vi "GetType.vi"(8 "error in (no error)":errorcluster, 11 "Set Output Value Msg":refnum<class "Set Output Value Msg.lvclass">) -> (0 "error out":errorcluster, 2 "Data Sample":variant, 3 "Set Output Value Msg":refnum<class "Set Output Value Msg.lvclass">)   [LabVIEW 2021, in "BNT_ULx.lvlib" / "Set Output Value Msg.lvclass"]
uses:
  Set Output Value Msg.lvclass
  Set Output Value Msg.lvclass/Set Output Value Msg.ctl
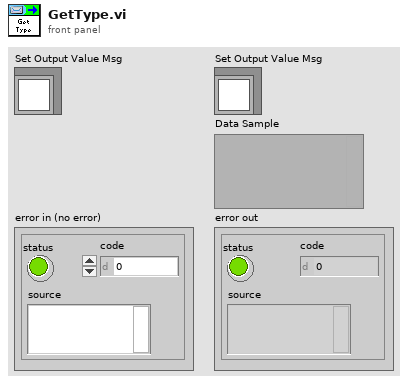
[diagram p1: front panel]
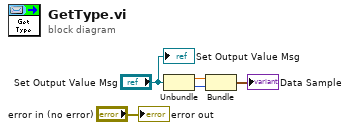
[diagram p0: block diagram]
diagram:
  n1 = Unbundle("Set Output Value Msg") -> (w2:dbl, w1:i32)
  n2 = Bundle("Value"=w2, "Channel"=w1) -> (→"Data Sample":cluster{"Value":dbl, "Channel":i32})  [unwired: 1 in]
  "error out" <- "error in (no error)"
  "Set Output Value Msg" <- "Set Output Value Msg"
